vi "Simple Get Multiple Buffers.vi"(0 "host uri":string, 1 "username":string, 2 "password":string, 5 "relative remote file uris":string[](array[string]), 11 "error in (no error)":errorcluster) -> (4 "data":string[](array[string]), 15 "error out":errorcluster)   [LabVIEW 2017, in "NI_WebDAV.lvlib"]
doc: "Returns a file or multiple files or the raw binary contents of a file or multiple files from a remote WebDAV server or target. You must manually select the polymorphic instance you want to use."
uses:
  <vilib>/WebDAVClient/NI_WebDAV.lvlib
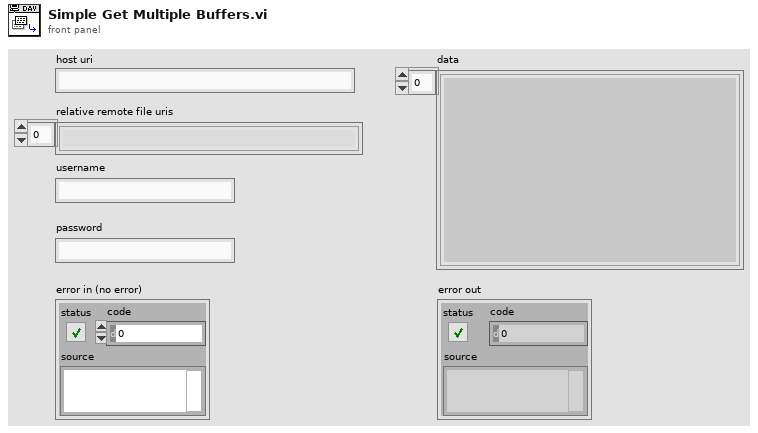
[diagram p1: front panel]
types:
  T1 = typedef "NI_WebDAV.lvlib/SessionHandle.ctl" = refnum<k1>
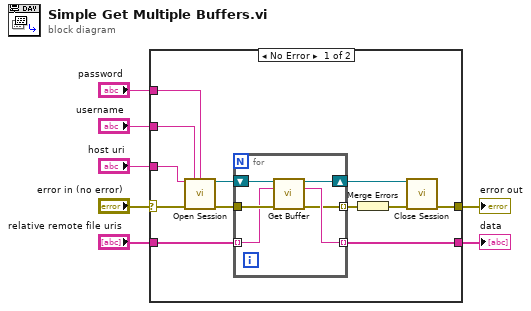
[diagram p0: block diagram]
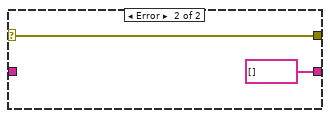
[diagram p2: hidden frame]
diagram:
  n1 = case shown="No Error" "error in (no error)" {
    selector: "error in (no error)" -> [w19 w27]
    tunnel: "host uri" -> [w18 _]
    tunnel: "username" -> [w17 _]
    tunnel: "password" -> [w16 _]
    tunnel: "relative remote file uris" -> [w14 _]
    tunnel: [w11 w27] -> w2
    tunnel: [w10 string[] []] -> w1
    frame No Error {
      n2 = call <vilib>:"Open Session.vi"("host uri prefix"=w18, "username"=w17, "password"=w16, "error in (no error)"=w19) -> ("session handle out"=w15:T1, "error out"=w9:errorcluster)  [unwired: 10 in]
      n3 = for {
        tunnel: w9 -> [w25]
        tunnel: w14 -> [w23] mode=indexing
        shift-right: [w22] -> w12
        shift-left: w15 -> [w24]
        tunnel: [w21] -> w10 mode=indexing
        tunnel: [w20] -> w8 mode=indexing
        n4 = call <vilib>:"Get Buffer.vi"("session handle"=w24, "relative uri"=w23, "error in (no error)"=w25) -> ("session handle out"=w22:T1, "data"=w21:string, "error out"=w20:errorcluster)  [unwired: 10 in]
      }
      n5 = Merge Errors(w8) -> (w13:errorcluster)
      n6 = call <vilib>:"Close Session.vi"("session handle"=w12, "error in (no error)"=w13) -> ("error out"=w11:errorcluster)  [unwired: 13 in]
    }
    frame Error {
    }
  }
  "error out" <- w2
  "data" <- w1
